vi "PH Sensor.vi"() -> (2 "SUGGESTED CROP":string, 3 "pH VALUE":dbl)   [LabVIEW 2013]
uses:
  <vilib>/myRIO/Instrument Drivers/Onboard IO/AI/vis/Smart Open.vi
  <vilib>/myRIO/Instrument Drivers/Onboard IO/AI/vis/Read.vi
  <vilib>/myRIO/Instrument Drivers/Onboard IO/AI/vis/Open.vi
  <vilib>/myRIO/Common/Instrument Driver Framework/myRIO v1.0/AI/vis/myRIO v1.1 Open AI.vi
  <vilib>/myRIO/Common/Instrument Driver Framework/Utilities/vis/Validate Channels.vi
  <vilib>/myRIO/Common/Instrument Driver Framework/myRIO v1.0/AI/vis/myRIO v1.0 Reserve AI.vi
  <vilib>/myRIO/Common/Instrument Driver Framework/myRIO v1.0/AI/vis/myRIO v1.0 Build MUX Configuration AI.vi
  <vilib>/myRIO/Common/Instrument Driver Framework/myRIO v1.0/Resource Manager/vis/myRIO v1.0 Reserve Channel List.vi
  <vilib>/myRIO/Common/Instrument Driver Framework/myRIO v1.0/Resource Manager/vis/myRIO v1.0 Reserve Channel.vi
  <vilib>/myRIO/Common/Instrument Driver Framework/myRIO v1.0/Resource Manager/vis/myRIO v1.0 Unreserve Channel.vi
  <vilib>/myRIO/Common/Instrument Driver Framework/myRIO v1.0/Resource Manager/vis/myRIO v1.0 Build Mutex Name.vi
  <vilib>/myRIO/Common/Instrument Driver Framework/myRIO v1.0/myRIO v1.1 Open.vi
  <vilib>/myRIO/Common/Instrument Driver Framework/myRIO v1.0/AI/vis/myRIO v1.0 Get Scaling Constants AI.vi
  <vilib>/Utility/VariantDataType/GetNumericInfo.vi
  <vilib>/Utility/error.llb/Error Cluster From Error Code.vi
  <vilib>/myRIO/Common/Instrument Driver Framework/Utilities/vis/IO Manager.vi
  <vilib>/myRIO/Common/Instrument Driver Framework/Utilities/vis/Configuration Manager.vi
  <vilib>/myRIO/Common/Instrument Driver Framework/myRIO v1.0/myRIO v1.0 Close.vi
  <vilib>/myRIO/Common/Instrument Driver Framework/myRIO v1.0/AI/vis/myRIO v1.0 Read AI.vi
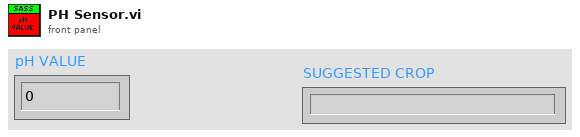
[diagram p1: front panel]
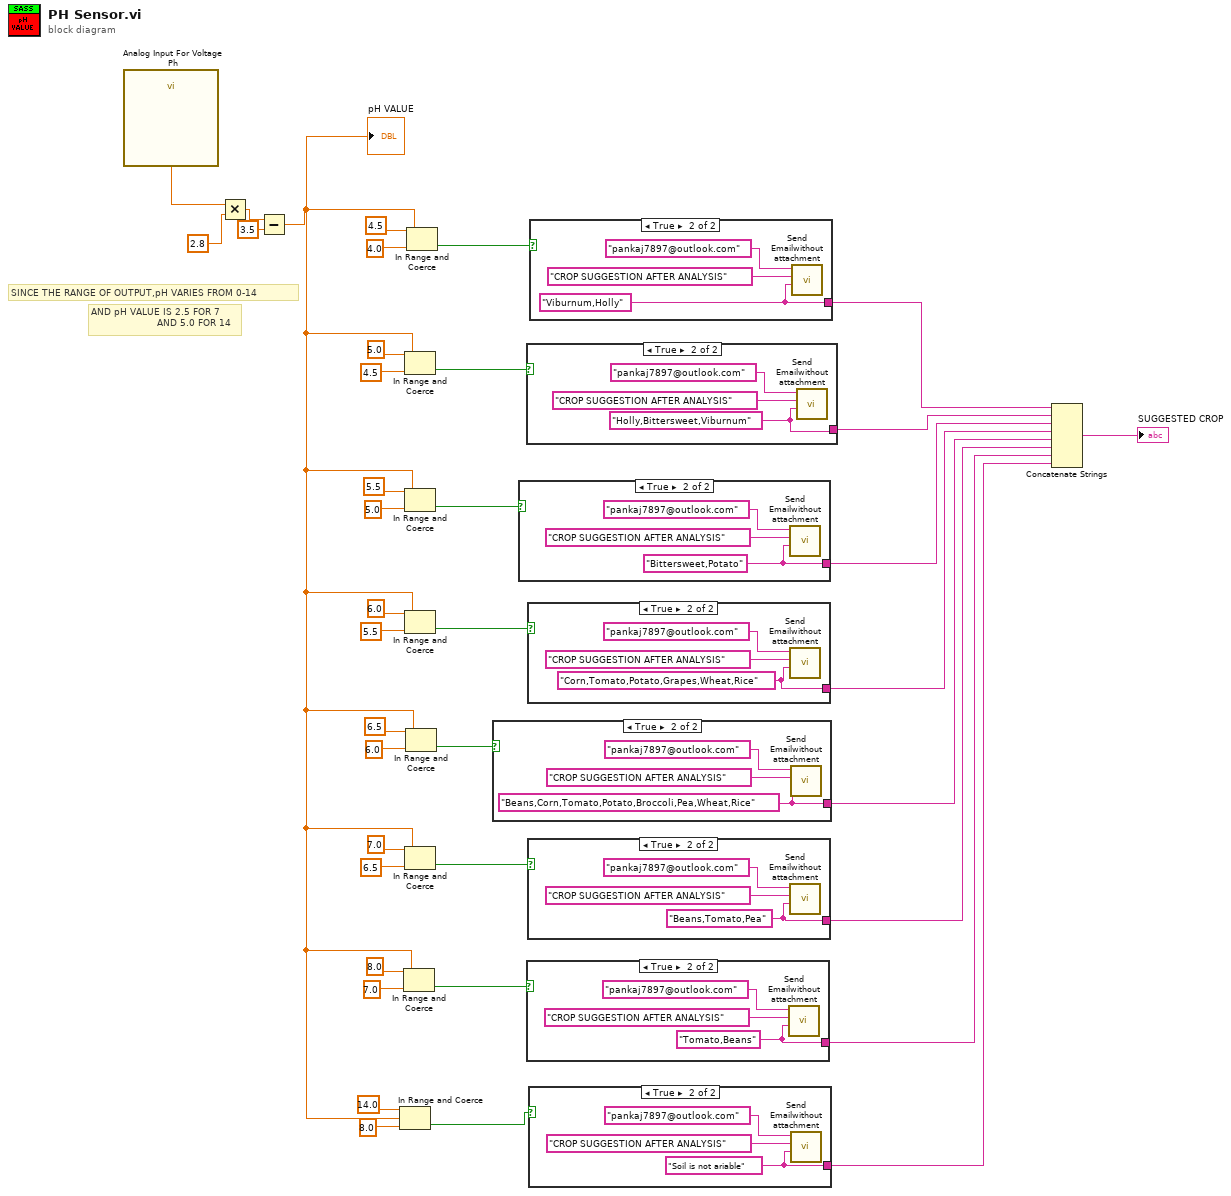
[diagram p0: block diagram]
diagram:
  # "AND pH VALUE IS 2.5 FOR 7\n                      AND 5.0 FOR 14"
  # "SINCE THE RANGE OF OUTPUT,pH VARIES FROM 0-14"
  n1 = call "Analog Input For Voltage Ph"() -> ("A/AI3 (Pin 9)"=w36:dbl)  [unwired: 26 in, 1 out]
  n2 = Multiply(x=w36, y=2.8 ("x*y")) -> (x*y=w15:dbl)
  n3 = Subtract(x=w15, y=3.5) -> (x-y=w10:dbl)
  "pH VALUE" <- w10
  n4 = In Range and Coerce(upper limit=14.0, x=w10, lower limit=8.0 ("upper limit")) -> (In Range?=w11:bool)  [unwired: 1 out]
  n5 = In Range and Coerce(upper limit=8.0, x=w10, lower limit=7.0 ("upper limit")) -> (In Range?=w16:bool)  [unwired: 1 out]
  n6 = In Range and Coerce(upper limit=5.0, x=w10, lower limit=4.5 ("upper limit")) -> (In Range?=w33:bool)  [unwired: 1 out]
  n7 = In Range and Coerce(upper limit=5.5, x=w10, lower limit=5.0 ("upper limit")) -> (In Range?=w28:bool)  [unwired: 1 out]
  n8 = In Range and Coerce(upper limit=6.0, x=w10, lower limit=5.5 ("upper limit")) -> (In Range?=w27:bool)  [unwired: 1 out]
  n9 = In Range and Coerce(upper limit=7.0, x=w10, lower limit=6.5 ("upper limit")) -> (In Range?=w21:bool)  [unwired: 1 out]
  n10 = In Range and Coerce(upper limit=6.5, x=w10, lower limit=6.0 ("upper limit")) -> (In Range?=w22:bool)  [unwired: 1 out]
  n11 = In Range and Coerce(upper limit=4.5, x=w10, lower limit=4.0 ("upper limit")) -> (In Range?=w34:bool)  [unwired: 1 out]
  n12 = case shown="True" w22 {
    tunnel: [_ w39] -> w5
    frame False {
    }
    frame True {
      w39 = "Beans,Corn,Tomato,Potato,Broccoli,Pea,Wheat,Rice" ("Message")
      n13 = call "Send Emailwithout attachment.vi"("To: 2"="pankaj7897@outlook.com", "Subject 2"="CROP SUGGESTION AFTER ANALYSIS", "Message 2"=w39) -> ()  [unwired: 8 in]
    }
  }
  n14 = case shown="True" w28 {
    tunnel: [_ w42] -> w7
    frame False {
    }
    frame True {
      w42 = "Bittersweet,Potato" ("Message")
      n15 = call "Send Emailwithout attachment.vi"("To: 2"="pankaj7897@outlook.com", "Subject 2"="CROP SUGGESTION AFTER ANALYSIS", "Message 2"=w42) -> ()  [unwired: 8 in]
    }
  }
  n16 = case shown="True" w33 {
    tunnel: [_ w45] -> w8
    frame False {
    }
    frame True {
      w45 = "Holly,Bittersweet,Viburnum" ("Message")
      n17 = call "Send Emailwithout attachment.vi"("To: 2"="pankaj7897@outlook.com", "Subject 2"="CROP SUGGESTION AFTER ANALYSIS", "Message 2"=w45) -> ()  [unwired: 8 in]
    }
  }
  n18 = case shown="True" w16 {
    tunnel: [_ w48] -> w4
    frame False {
    }
    frame True {
      w48 = "Tomato,Beans" ("Message")
      n19 = call "Send Emailwithout attachment.vi"("To: 2"="pankaj7897@outlook.com", "Subject 2"="CROP SUGGESTION AFTER ANALYSIS", "Message 2"=w48) -> ()  [unwired: 8 in]
    }
  }
  n20 = case shown="True" w27 {
    tunnel: [_ w51] -> w6
    frame False {
    }
    frame True {
      w51 = "Corn,Tomato,Potato,Grapes,Wheat,Rice" ("Message")
      n21 = call "Send Emailwithout attachment.vi"("To: 2"="pankaj7897@outlook.com", "Subject 2"="CROP SUGGESTION AFTER ANALYSIS", "Message 2"=w51) -> ()  [unwired: 8 in]
    }
  }
  n22 = case shown="True" w21 {
    tunnel: [_ w54] -> w2
    frame False {
    }
    frame True {
      w54 = "Beans,Tomato,Pea" ("Message")
      n23 = call "Send Emailwithout attachment.vi"("To: 2"="pankaj7897@outlook.com", "Subject 2"="CROP SUGGESTION AFTER ANALYSIS", "Message 2"=w54) -> ()  [unwired: 8 in]
    }
  }
  n24 = case shown="True" w11 {
    tunnel: [_ w57] -> w3
    frame False {
    }
    frame True {
      w57 = "Soil is not ariable" ("Message")
      n25 = call "Send Emailwithout attachment.vi"("To: 2"="pankaj7897@outlook.com", "Subject 2"="CROP SUGGESTION AFTER ANALYSIS", "Message 2"=w57) -> ()  [unwired: 8 in]
    }
  }
  n26 = case shown="True" w34 {
    tunnel: [_ w60] -> w9
    frame False {
    }
    frame True {
      w60 = "Viburnum,Holly" ("Message")
      n27 = call "Send Emailwithout attachment.vi"("To: 2"="pankaj7897@outlook.com", "Subject 2"="CROP SUGGESTION AFTER ANALYSIS", "Message 2"=w60) -> ()  [unwired: 8 in]
    }
  }
  n28 = Concatenate Strings(w9, w8, w7, w6, w5, w2, w4, w3) -> (→"SUGGESTED CROP":string)
